vi "GetIsBig.vi"(8 "Error In":errorcluster, 11 "reference in":refnum<class "12_Cave.lvclass">) -> (0 "Error Out":errorcluster, 2 "Is Big":bool, 3 "reference out":refnum<class "12_Cave.lvclass">)   [LabVIEW 2020, in "12_Cave.lvclass"]
uses:
  12_Cave.lvclass
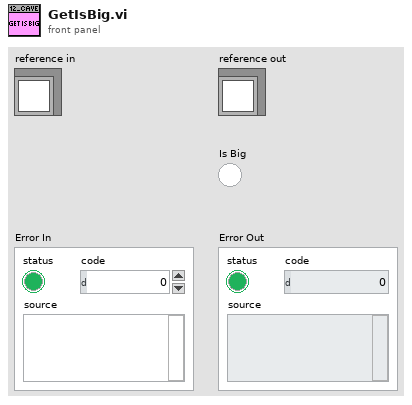
[diagram p1: front panel]
types:
  T1 = typedef "12_Cave.lvclass/ObjectAttributes.ctl" = cluster{"Neighbours":refnum<class "12_Cave.lvclass">[], "Is Big":bool, "Name":string}
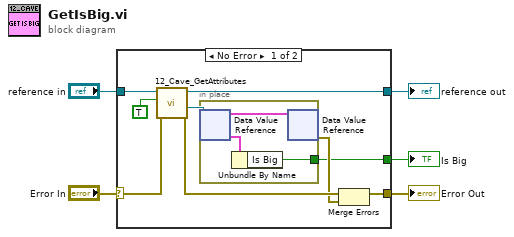
[diagram p0: block diagram]
diagram:
  n1 = case shown="No Error" "Error In" {
    selector: "Error In" -> [w14 w18]
    tunnel: [w12 w18] -> w4
    tunnel: [w9 w17] -> w2
    tunnel: "reference in" -> [w10 w17]
    tunnel: [w6 _] -> w1
    frame No Error {
      n2 = call "12_Cave_GetAttributes.vi"("error in (no error)"=w14, "OnlyGetDvrReference(False)"=TRUE, "reference in"=w10) -> ("error out"=w13:errorcluster, "DataRef"=w7:refnum<data-value>, "reference out"=w9:refnum<class "12_Cave.lvclass">)  [unwired: 5 in, 1 out]
      n3 = in-place {
        in-place-border: [w16] -> w6
        n4 = in-place-dvr #1(w7) -> (w15:T1)  [unwired: 1 out]
        n5 = Unbundle By Name(w15) -> ("Is Big"=w16:bool)
        n6 = in-place-dvr #1(w15) -> (w11:errorcluster)  [unwired: 1 out]
      }
      n7 = Merge Errors(w13, w11) -> (w12:errorcluster)
    }
    frame Error {
    }
  }
  "Error Out" <- w4
  "reference out" <- w2
  "Is Big" <- w1
